vi "Get Instrument Dependencies.vi"(8 "error in (no error)":errorcluster, 11 "Instrument in":refnum<class "Instrument.lvclass">) -> (0 "error out":errorcluster, 2 "Dependencies":T1, 3 "SMO out":refnum<class "Instrument.lvclass">)   [LabVIEW 2016, in "Instrument.lvclass"]
uses:
  Instrument.lvclass
  levylab_util_remote/src/SMOs/RemoteControl/RemoteControl.lvclass
  Logger/Logger.lvclass
  C:/Program Files (x86)/National Instruments/LabVIEW 2016/vi.lib/JKI/JKI SMO/SMO/SMO.lvclass
  <vilib>/JKI/JKI SMO/SMO/SMO.lvclass
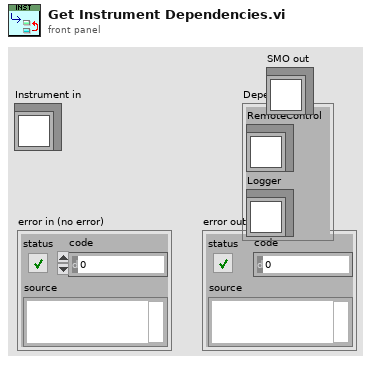
[diagram p1: front panel]
types:
  T1 = cluster{"RemoteControl":refnum<class "RemoteControl.lvclass">, "Logger":refnum<class "Logger.lvclass">}
  T2 = cluster{"RemoteControl.lvclass":refnum<class "RemoteControl.lvclass">, "Logger.lvclass":refnum<class "Logger.lvclass">}
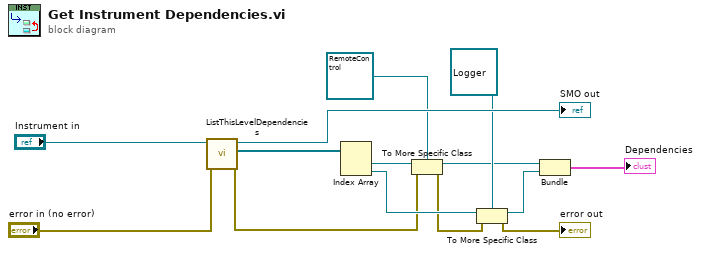
[diagram p0: block diagram]
diagram:
  n1 = call <vilib>:"ListThisLevelDependencies.vi"("error in (no error)"="error in (no error)", "SMO in"="Instrument in") -> ("error out"=w8:errorcluster, "[My Dependencies]"=w13:refnum<class "SMO.lvclass">[], "SMO out"=→"SMO out":refnum<class "Instrument.lvclass">)  [unwired: 7 in]
  n2 = Index Array(array=w13) -> (element #1=w14:refnum<class "SMO.lvclass">, element #2=w9:refnum<class "SMO.lvclass">)  [unwired: 2 in]
  n3 = To More Specific Class(target class=refnum<class "RemoteControl.lvclass"> refnum ("RemoteControl.lvclass"), reference=w14, error in=w8) -> (specific class reference=w3:refnum<class "RemoteControl.lvclass">, error out=w7:errorcluster)
  n4 = To More Specific Class(target class=refnum<class "Logger.lvclass"> refnum ("Logger.lvclass"), reference=w9, error in=w7) -> (specific class reference=w2:refnum<class "Logger.lvclass">, error out=→"error out":errorcluster)
  n5 = Bundle("RemoteControl.lvclass"=w3, "Logger.lvclass"=w2) -> (→"Dependencies":T2)  [unwired: 1 in]
